vi "L-STF Autocorrelation.vi"(9 "input valid":bool, 10 "sample":T2) -> (1 "output valid":bool, 2 "auto correlation":T1)   [LabVIEW 2020]
uses:
  <vilib>/rvi/FXPMathLib/basic elements/FxpDiscreteDelay/XNode/nifxpmath_DiscreteDelay.xnode
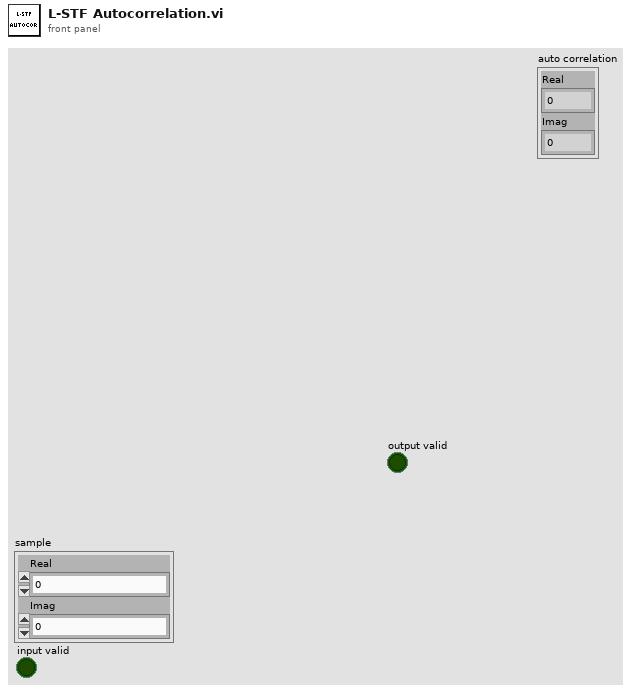
[diagram p1: front panel]
types:
  T1 = cluster{"Real":fxp<+/-,42,16>, "Imag":fxp<+/-,42,16>}
  T2 = cluster{"Real":fxp<+/-,16,3>, "Imag":fxp<+/-,16,3>}
  T3 = cluster{"EIFS":u32, "ACK timeout":u32, "CTS timeout":u32, "aRxPHYStartDelay":u32, "Frame control field length":u16, "Duration/ID field length":u16, "aSlotTime":u32, "aSIFSTime":u32, "PIFS":u32, "DIFS":u32, "Address field length":u16, "Sequence control field length":u16, "QoS control field length":u16, "HT control field length":u16, "FCS field length":u16, "MPDU delimiter length":u16, "MPDU delimiter signature":u16, "Max MPDU buffer length":u16, "timestamp steps / mks":u32, "L-STF periods / L-STF":u8, "sample / L-STF period":u8, "T_SIGNAL":u16, "N_tail":u16, "N_service":u16, "N_ES":u16, "N_SS":u16, "m_STBC":u16, "T_VHTSIGB":u16, "T_VHTPREAMBLE":u16, "T_VHTSIGA":u16, "T_LSIG":u16, "T_LEGPREAMBLE":u16, "NOFDM_VHTSIGB":u16, "T_SYM":u16, "T_SYML":u16, "NOFDM_PREAMBLE":u16, "NOFDM_SIGNAL":u16, "T_PREAMBLE":u16, "NOFDM_LEGPREAMBLE":u16, "NOFDM_VHTPREAMBLE":u16, "NOFDM_VHTSIGA":u16, "NOFDM_LSIG":u16, "NOFDM_VHTPREAMBLE 2":u16, "NOFDM_LSIG 2":u16}
  T4 = cluster{"Real":fxp<+/-,33,7>, "Imag":fxp<+/-,33,7>}
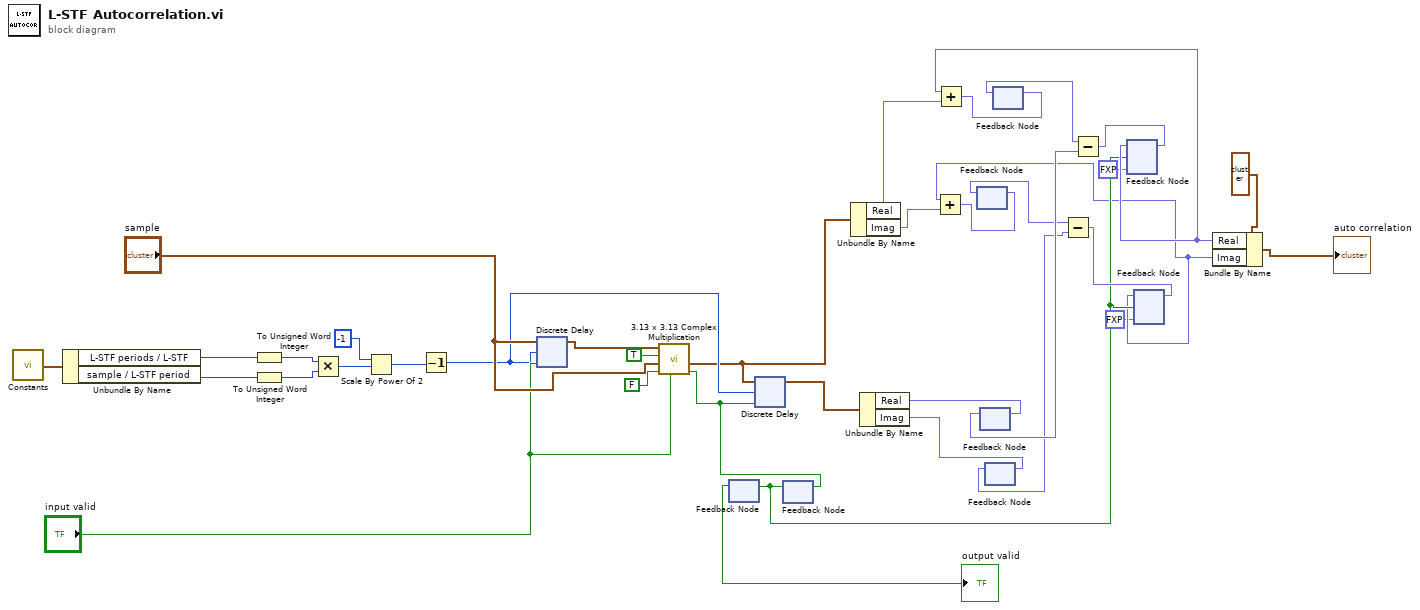
[diagram p0: block diagram]
diagram:
  n1 = call "Constants.vi"() -> ("output cluster"=w37:T3)  [unwired: 11 in]
  n2 = Unbundle By Name(w37) -> ("L-STF periods / L-STF"=w36:u8, "sample / L-STF period"=w35:u8)
  n3 = To Unsigned Word Integer(number=w36) -> (unsigned 16bit integer=w34:u16)
  n4 = To Unsigned Word Integer(number=w35) -> (unsigned 16bit integer=w33:u16)
  n5 = Multiply(x=w34, y=w33) -> (x*y=w32:u16)
  n6 = Scale By Power Of 2(n=i16 -1, x=w32) -> (x*2^n=w31:u16)
  n7 = Decrement(x=w31) -> (x-1=w24:u16)
  n8 = xnode ("Discrete Delay")("D"="sample", "n-1[0..319]"=w24, "enable"="input valid") -> ("Q"=w29:T2)
  n9 = call "3.13 x 3.13 Complex Multiplication.vi"("input valid"="input valid", "conjugate B"=FALSE, "B"="sample", "conjugate A"=TRUE, "A"=w29) -> ("output valid"=w23:bool, "product"=w20:T4)  [unwired: 5 in]
  n10 = feedback #1() -> (→"output valid":bool)  [unwired: 1 in]
  n11 = xnode ("Discrete Delay")("D"=w20, "n-1[0..319]"=w24, "enable"=w23) -> ("Q"=w19:T4)
  n12 = feedback #2() -> (w4:bool)  [unwired: 1 in]
  n13 = feedback-in #1(w4) -> ()
  n14 = feedback-in #2(w23) -> ()
  n15 = Unbundle By Name(w20) -> ("Real"=w18:fxp<+/-,33,7>, "Imag"=w10:fxp<+/-,33,7>)
  n16 = Unbundle By Name(w19) -> ("Real"=w12:fxp<+/-,33,7>, "Imag"=w7:fxp<+/-,33,7>)
  n17 = feedback #3() -> (w8:fxp<+/-,43,17>)  [unwired: 1 in]
  n18 = feedback #4() -> (w13:fxp<+/-,33,7>)  [unwired: 1 in]
  n19 = feedback-in #4(w12) -> ()
  n20 = feedback #5() -> (w6:fxp<+/-,33,7>)  [unwired: 1 in]
  n21 = feedback-in #5(w7) -> ()
  n22 = feedback #6() -> (w17:fxp<+/-,43,17>)  [unwired: 1 in]
  n23 = Subtract(x=w8, y=w6) -> (x-y=w5:fxp<+/-,42,16>)
  n24 = Subtract(x=w17, y=w13) -> (x-y=w16:fxp<+/-,42,16>)
  n25 = feedback #7(fxp<+/-,42,16> 0.0) -> (w11:fxp<+/-,42,16>)
  n26 = Add(x=w11, y=w18) -> (x+y=w21:fxp<+/-,43,17>)
  n27 = feedback-in #6(w21) -> ()
  n28 = feedback-in #7(w16, w4) -> ()
  n29 = feedback #8(fxp<+/-,42,16> 0.0) -> (w3:fxp<+/-,42,16>)
  n30 = Add(x=w3, y=w10) -> (x+y=w9:fxp<+/-,43,17>)
  n31 = feedback-in #3(w9) -> ()
  n32 = feedback-in #8(w5, w4) -> ()
  n33 = Bundle By Name(cluster=T1 {"Real"=0.0, "Imag"=0.0} ("auto correlation"), "Real"=w11, "Imag"=w3) -> (→"auto correlation":T1)
